vi "getCost.vi"(8 "error in (no error)":errorcluster, 11 "Milk in":refnum<class "Milk.lvclass">) -> (0 "error out":errorcluster, 2 "cost":dbl, 3 "Milk out":refnum<class "Milk.lvclass">)   [LabVIEW 2017, in "Milk.lvclass"]
uses:
  Milk.lvclass
  CondimentDecorator/CondimentDecorator.lvclass
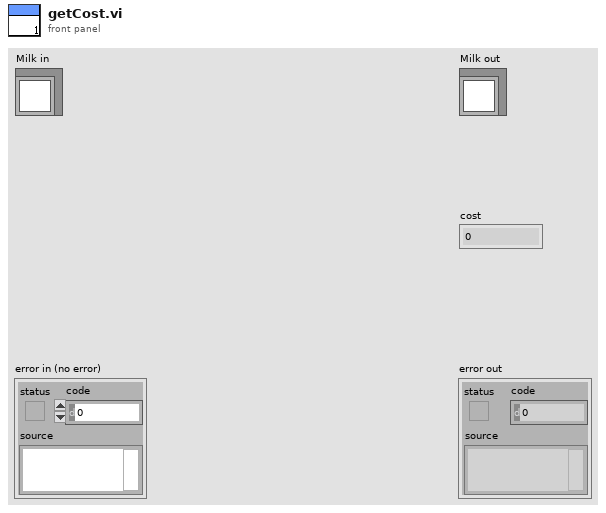
[diagram p1: front panel]
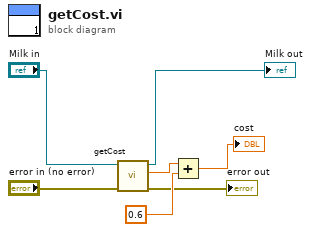
[diagram p0: block diagram]
diagram:
  n1 = call-parent "getCost.vi"("error in (no error)"="error in (no error)", "CondimentDecorator in"="Milk in") -> ("error out"=→"error out":errorcluster, "cost"=w1:dbl, "CondimentDecorator out"=→"Milk out":refnum<class "Milk.lvclass">)  [unwired: 7 in]
  n2 = Add(x=w1, y=0.6) -> (x+y=→"cost":dbl)
